vi "ISO8601Timestamp.vi"() -> (1 "date/time string":string)   [LabVIEW 2018]
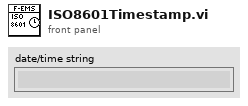
[diagram p1: front panel]
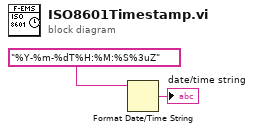
[diagram p0: block diagram]
diagram:
  n1 = Format Date/Time String(time format string (%c)="%Y-%m-%dT%H:%M:%S%3uZ") -> (date/time string=→"date/time string":string)  [unwired: 2 in]
